vi "CE14.Open.handshake.vi"(8 "error in (no error)":errorcluster, 11 "CE14 cluster":T1={"VISA resource name"="COM12", "baudrate"=300}) -> (0 "error out":errorcluster, 3 "CE14 cluster":T1={"VISA resource name"="", "baudrate"=300})   [LabVIEW 2018]
uses:
  type defs/CE14_cluster.ctl
  <vilib>/Instr/_visa.llb/VISA Configure Serial Port (Instr).vi
  CE14_Globals.vi
  CE14_eMIC.lvlib
panel:
  out "x-y":dbl format="%.12f"
  out "return count 2":u32
  out "4800_2":string
  out "4800_1":string
  out "300_1":string
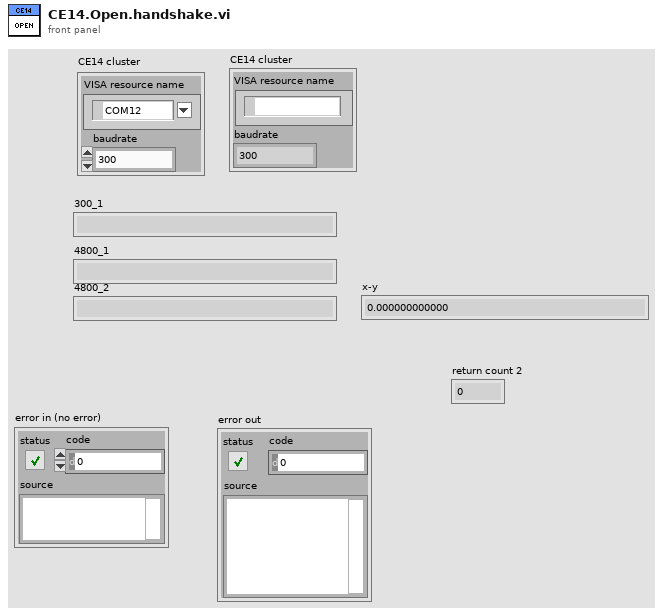
[diagram p1: front panel]
types:
  T1 = typedef "CE14_eMIC.lvlib/CE14_cluster.ctl" = cluster{"VISA resource name":refnum<visa-resource-name>, "baudrate":u32}
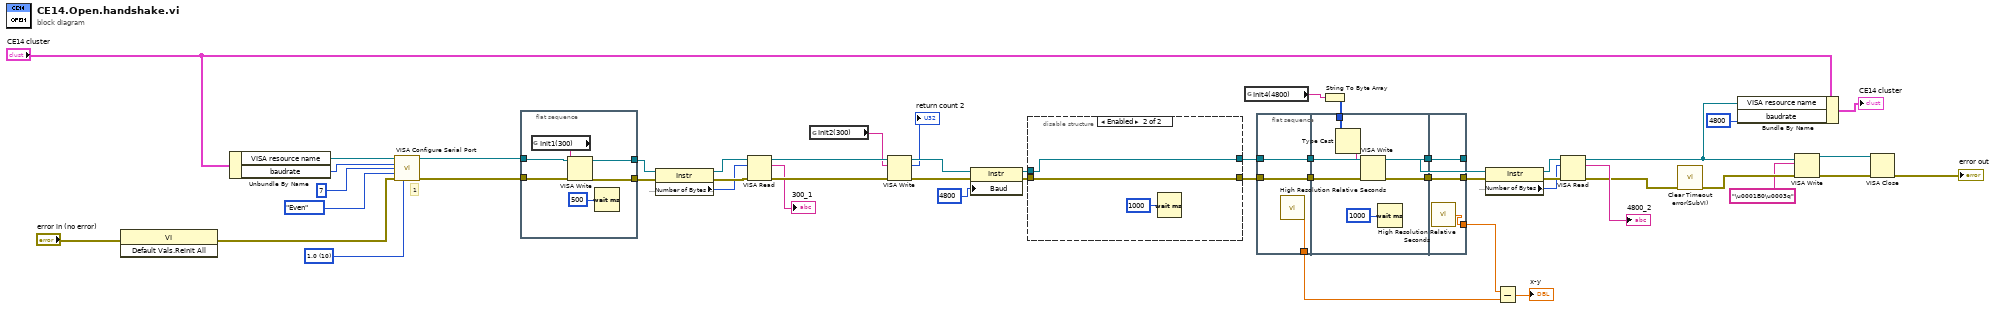
[diagram p0: block diagram]
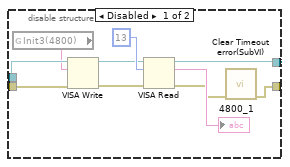
[diagram p2: hidden frame]
diagram:
  w47 = u16 10 items=["1.0"=10, "1.5"=15, "2.0"=20] ("stop bits (10: 1 bit)")
  # "1"
  n1 = invoke class="VI" method="Default Vals.Reinit All"(error in="error in (no error)") -> (error out=w23:errorcluster)  [unwired: 2 in, 2 out]
  n2 = Unbundle By Name("CE14 cluster") -> ("VISA resource name"=w51:refnum<visa-resource-name>, "baudrate"=w50:u32)
  n3 = call-poly "VISA Configure Serial Port"("VISA resource name"=w51, "baud rate (9600)"=w50, "data bits (8)"=u16 7, "parity (0:none)"=enum16{"None", "Odd", "Even", "Mark", "Space"}."Even", "error in (no error)"=w23, "stop bits (10: 1 bit)"=w47) -> ("VISA resource name out"=w2:refnum<visa-resource-name>, "error out"=w1:errorcluster)  [unwired: 8 in]
  n4 = flat-sequence {
    tunnel: [w57] -> w46
    tunnel: [w56] -> w45
    tunnel: w1 -> [w55]
    tunnel: w2 -> [w54]
    frame #0 {
      n5 = global read "CE14_Globals.vi" "Init1(300)"() -> (w53:string)
      n6 = VISA Write(VISA resource name=w54, write buffer=w53, error in (no error)=w55) -> (VISA resource name out=w56:refnum<visa-resource-name>, error out=w57:errorcluster)  [unwired: 1 out]
      n7 = Wait (ms)(milliseconds to wait=u32 500) -> ()  [unwired: 1 out]
    }
  }
  n8 = property class="Instr"(reference=w45, error in=w46) -> (reference out=w43:refnum<visa-resource-name>, error out=w44:errorcluster, "Serial Settings:Number of Bytes at Serial Port"=w42:u32)
  n9 = VISA Read(VISA resource name=w43, byte count=w42, error in (no error)=w44) -> (VISA resource name out=w39:refnum<visa-resource-name>, read buffer=→"300_1":string, error out=w40:errorcluster)  [unwired: 1 out]
  n10 = global read "CE14_Globals.vi" "Init2(300)"() -> (w22:string)
  n11 = VISA Write(VISA resource name=w39, write buffer=w22, error in (no error)=w40) -> (VISA resource name out=w30:refnum<visa-resource-name>, return count=→"return count 2":u32, error out=w29:errorcluster)
  n12 = property class="Instr"(reference=w30, error in=w29, "Baud"=u32 4800 ("baud rate (9600)")) -> (reference out=w35:refnum<visa-resource-name>, error out=w34:errorcluster)
  n13 = disable-structure shown="Enabled" {
    disable-tunnel: w35 -> [w67 w69]
    disable-tunnel: w34 -> [w66 w70]
    disable-tunnel: [w65 w69] -> w33
    disable-tunnel: [w59 w70] -> w26
    frame Disabled {
      n14 = global read "CE14_Globals.vi" "Init3(4800)"() -> (w58:string)
      n15 = VISA Write(VISA resource name=w67, write buffer=w58, error in (no error)=w66) -> (VISA resource name out=w61:refnum<visa-resource-name>, error out=w63:errorcluster)  [unwired: 1 out]
      n16 = VISA Read(VISA resource name=w61, byte count=u32 13, error in (no error)=w63) -> (VISA resource name out=w65:refnum<visa-resource-name>, read buffer=→"4800_1":string, error out=w60:errorcluster)  [unwired: 1 out]
      n17 = call "Clear Timeout error(SubVI).vi"("error in (no error)"=w60) -> ("error out"=w59:errorcluster)  [unwired: 10 in]
    }
    frame Enabled {
      n18 = Wait (ms)(milliseconds to wait=u32 1000) -> ()  [unwired: 1 out]
    }
  }
  n19 = global read "CE14_Globals.vi" "Init4(4800)"() -> (w4:string)
  n20 = flat-sequence {
    tunnel: w26 -> [w72]
    tunnel: w33 -> [w73]
    tunnel: [w73] -> w11
    tunnel: [w72] -> w10
    tunnel: [w71] -> w6
    tunnel: w11 -> [w80]
    tunnel: w10 -> [w77]
    tunnel: [w79] -> w9
    tunnel: [w78] -> w8
    tunnel: w3 -> [w75]
    tunnel: [w82] -> w27
    tunnel: [w83] -> w14
    tunnel: w9 -> [w83]
    tunnel: w8 -> [w82]
    tunnel: [w81] -> w7
    frame #0 {
      n21 = call <vilib>:"High Resolution Relative Seconds.vi"() -> ("relative seconds"=w71:dbl)
    }
    frame #1 {
      n22 = Type Cast(x=w75) -> (*(type *) &x=w74:string)  [unwired: 1 in]
      n23 = VISA Write(VISA resource name=w80, write buffer=w74, error in (no error)=w77) -> (VISA resource name out=w79:refnum<visa-resource-name>, error out=w78:errorcluster)  [unwired: 1 out]
      n24 = Wait (ms)(milliseconds to wait=u32 1000) -> ()  [unwired: 1 out]
    }
    frame #2 {
      n25 = call <vilib>:"High Resolution Relative Seconds.vi"() -> ("relative seconds"=w81:dbl)
    }
  }
  n26 = String To Byte Array(string=w4) -> (unsigned byte array=w3:u8[])
  n27 = property class="Instr"(reference=w14, error in=w27) -> (reference out=w13:refnum<visa-resource-name>, error out=w15:errorcluster, "Serial Settings:Number of Bytes at Serial Port"=w12:u32)
  n28 = Subtract(x=w7, y=w6) -> (x-y=→"x-y":dbl)
  n29 = VISA Read(VISA resource name=w13, byte count=w12, error in (no error)=w15) -> (VISA resource name out=w19:refnum<visa-resource-name>, read buffer=→"4800_2":string, error out=w25:errorcluster)  [unwired: 1 out]
  n30 = call "Clear Timeout error(SubVI).vi"("error in (no error)"=w25) -> ("error out"=w18:errorcluster)  [unwired: 10 in]
  n31 = Bundle By Name(cluster="CE14 cluster", "VISA resource name"=w19, "baudrate"=u32 4800) -> (→"CE14 cluster":T1)
  n32 = VISA Write(VISA resource name=w19, write buffer="\u0001B0\u0003q", error in (no error)=w18) -> (VISA resource name out=w20:refnum<visa-resource-name>, error out=w21:errorcluster)  [unwired: 1 out]
  n33 = VISA Close(VISA resource name=w20, error in (no error)=w21) -> (error out=→"error out":errorcluster)
